vi "Map the Signals and Frames.vi"(8 "error in":errorcluster, 11 "References":T1) -> (0 "error out":errorcluster)   [LabVIEW 2025, in "CAN-LIN Raw Bus Capture UI.lvlib"]
uses:
  CAN-LIN Raw Bus Capture UI.lvlib
  <vilib>/xnet/xnet.llb/XNET Create Session (Conversion).vi
  <resource>/objmgr/xnet.rc
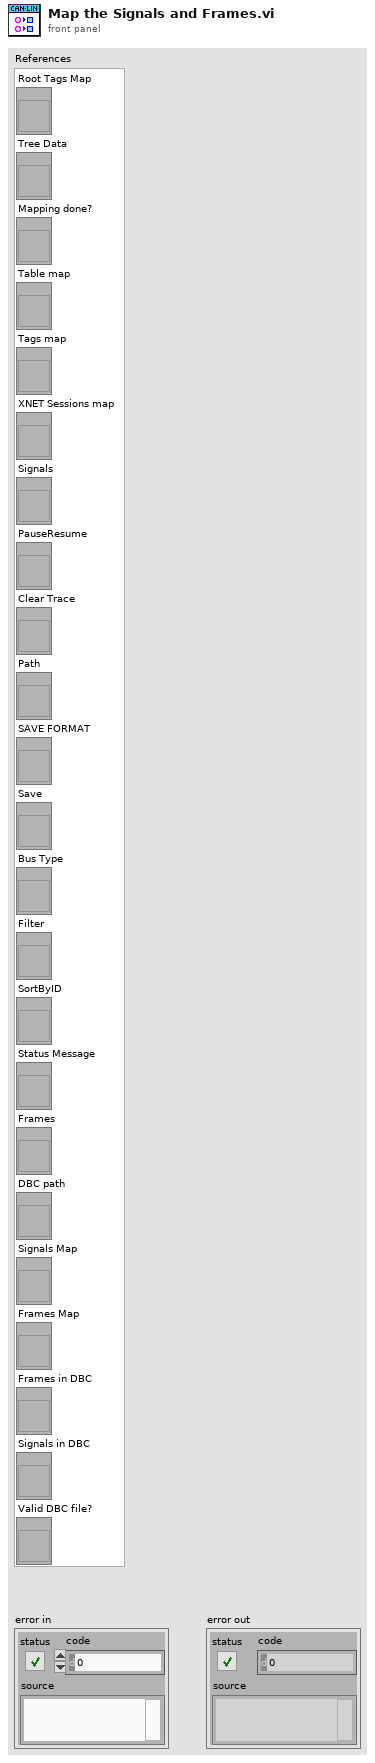
[diagram p1: front panel]
types:
  T1 = cluster{"Root Tags Map":refnum<vi>, "Tree Data":refnum<vi>, "Mapping done?":refnum<vi>, "Table map":refnum<vi>, "Tags map":refnum<vi>, "XNET Sessions map":refnum<vi>, "Signals":refnum<vi>, "PauseResume":refnum<vi>, "Clear Trace":refnum<vi>, "Path":refnum<vi>, "SAVE FORMAT":refnum<vi>, "Save":refnum<vi>, "Bus Type":refnum<vi>, "Filter":refnum<vi>, "SortByID":refnum<vi>, "Status Message":refnum<vi>, "Frames":refnum<vi>, "DBC path":refnum<vi>, "Signals Map":refnum<vi>, "Frames Map":refnum<vi>, "Frames in DBC":refnum<vi>, "Signals in DBC":refnum<vi>, "Valid DBC file?":refnum<vi>}
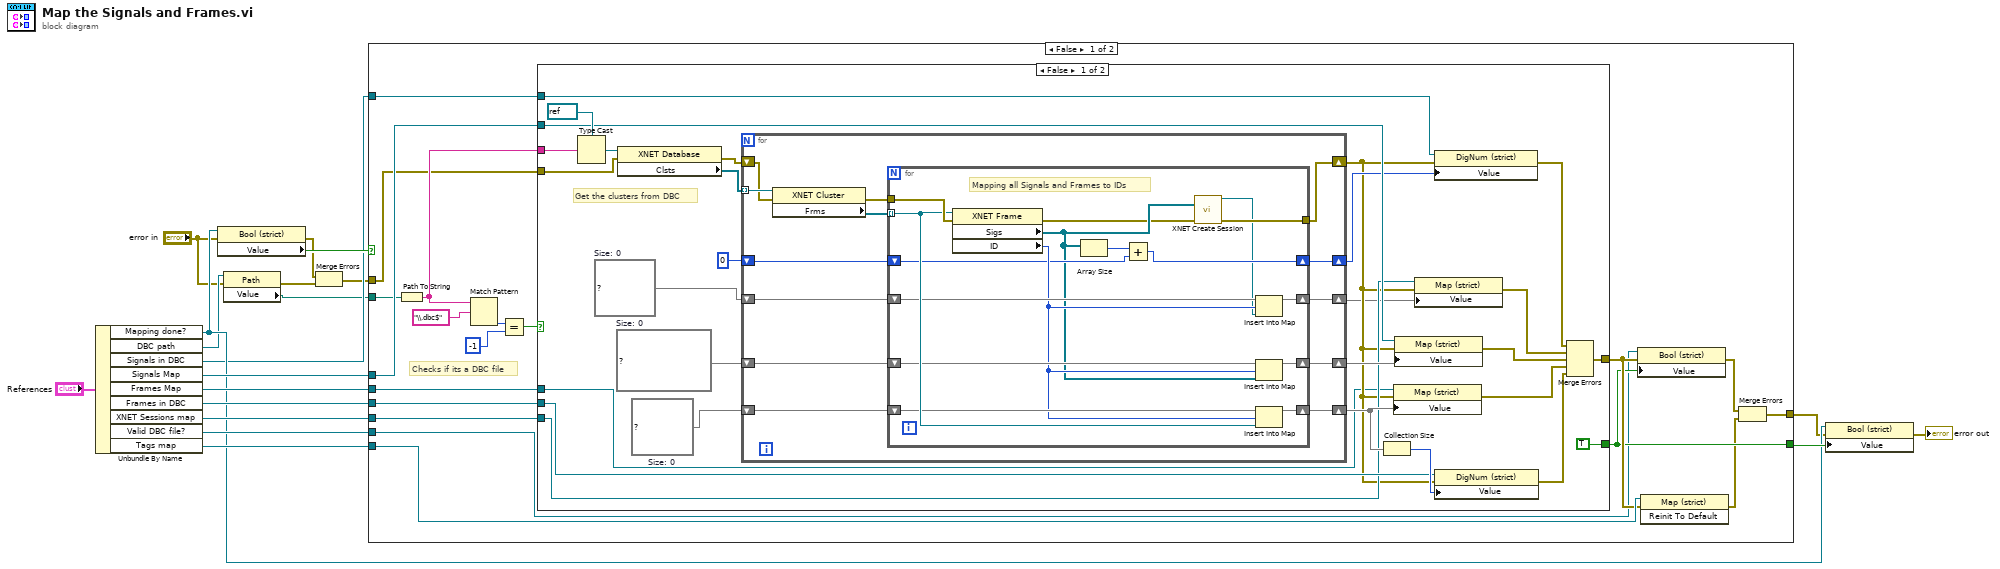
[diagram p0: block diagram]
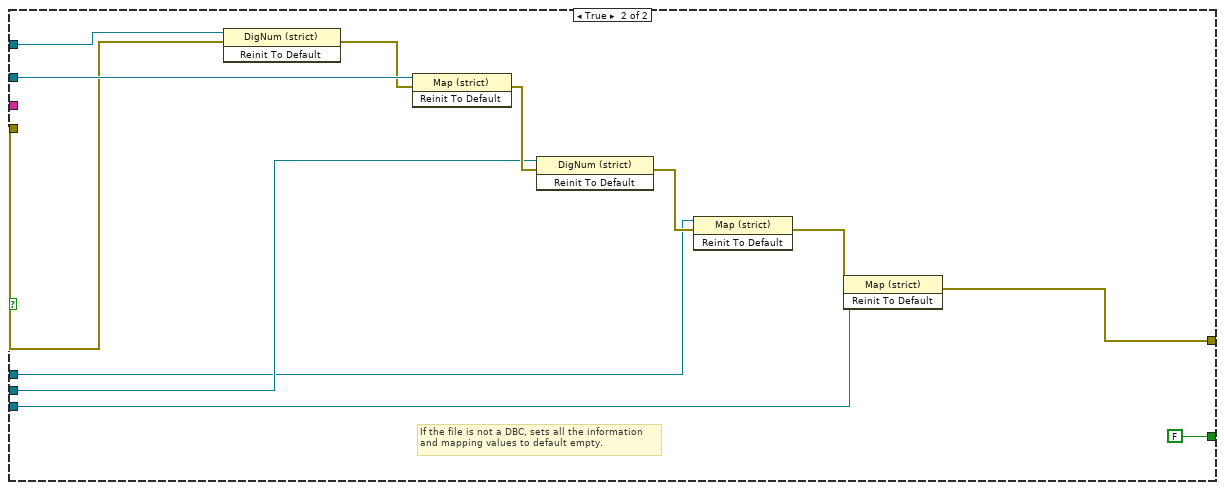
[diagram p2: hidden frame]
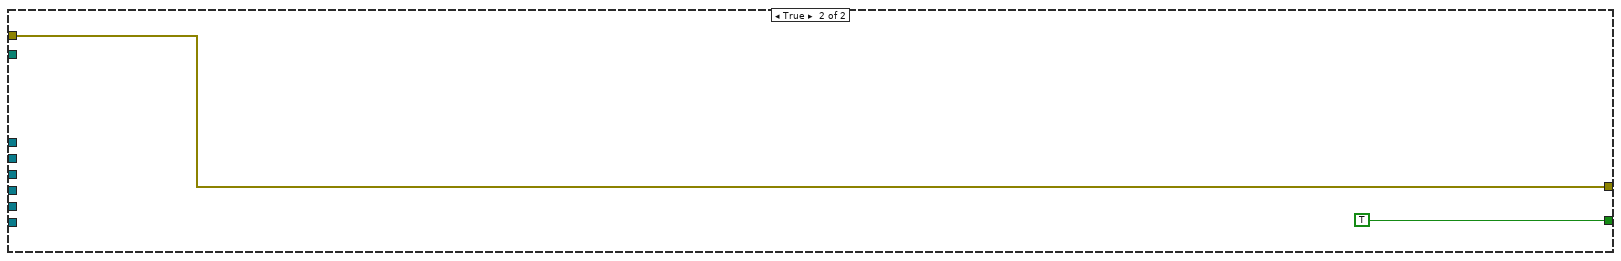
[diagram p3: hidden frame]
diagram:
  n1 = Unbundle By Name("References") -> ("Mapping done?"=w11:refnum<vi>, "DBC path"=w7:refnum<vi>, "Signals in DBC"=w8:refnum<vi>, "Signals Map"=w16:refnum<vi>, "Frames Map"=w19:refnum<vi>, "Frames in DBC"=w18:refnum<vi>, "XNET Sessions map"=w17:refnum<vi>, "Valid DBC file?"=w14:refnum<vi>, "Tags map"=w15:refnum<vi>)
  n2 = property class="Bool (strict)"(reference=w11, error in="error in") -> (error out=w3:errorcluster, "Value"=w13:bool)  [unwired: 1 out]
  n3 = property class="Path"(reference=w7, error in="error in") -> (error out=w5:errorcluster, "Value"=w2:path)  [unwired: 1 out]
  n4 = Merge Errors(w3, w5) -> (w4:errorcluster)
  n5 = case shown="False" w13 {
    tunnel: [w24 w108] -> w10
    tunnel: w4 -> [w20 w108]
    tunnel: [w27 TRUE ("Mapping done?")] -> w12
    tunnel: w19 -> [w37 _]
    tunnel: w16 -> [w38 _]
    tunnel: w18 -> [w31 _]
    tunnel: w8 -> [w30 _]
    tunnel: w17 -> [w23 _]
    tunnel: w14 -> [w22 _]
    tunnel: w15 -> [w29 _]
    tunnel: w2 -> [w21 _]
    frame False {
      # "Checks if its a DBC file"
      n6 = Path To String(path=w21) -> (string=w35:string)
      n7 = Match Pattern(string=w35, regular expression="\\.dbc$") -> (offset past match=w34:i32)  [unwired: 1 in, 3 out]
      n8 = Equal?(x=w34, y=-1) -> (x = y?=w32:bool)
      n9 = case shown="False" w32 {
        tunnel: w20 -> [w60 w100]
        tunnel: [TRUE ("Mapping done?") FALSE ("Mapping done?")] -> w27
        tunnel: w38 -> [w58 w102]
        tunnel: w37 -> [w39 w97]
        tunnel: [w55 w105] -> w28
        tunnel: w35 -> [w54 _]
        tunnel: w31 -> [w50 w98]
        tunnel: w30 -> [w46 w96]
        tunnel: w23 -> [w45 w106]
        frame False {
          w42 = map{u32, refnum<k21>} {}  # Size: 0
          w61 = map{u32, refnum<k21>} {}  # Size: 0
          w62 = map{u32, refnum<k21>[]} {}  # Size: 0
          # "Get the clusters from DBC"
          n10 = Type Cast(type=refnum<k21> refnum ("XNET Database"), x=w54) -> (*(type *) &x=w65:refnum<k21>)
          n11 = property class="XNET Database"(reference=w65, error in=w60) -> (error out=w66:errorcluster, "Clsts"=w64:refnum<k21>[])  [unwired: 1 out]
          n12 = for {
            tunnel: w64 -> [w79] mode=indexing
            shift-right: [w74] -> w52
            shift-left: w62 -> [w73]
            shift-right: [w72] -> w53
            shift-left: w61 -> [w71]
            shift-right: [w69] -> w47
            shift-left: 0 -> [w70]
            shift-right: [w75] -> w44
            shift-left: w66 -> [w77]
            shift-right: [w67] -> w40
            shift-left: w42 -> [w68]
            n13 = property class="XNET Cluster"(reference=w79, error in=w77) -> (error out=w76:errorcluster, "Frms"=w78:refnum<k21>[])  [unwired: 1 out]
            n14 = for {
              tunnel: w78 -> [w94] mode=indexing
              tunnel: w76 -> [w95]
              tunnel: [w81] -> w75
              shift-right: [w93] -> w74
              shift-left: w73 -> [w92]
              shift-right: [w91] -> w72
              shift-left: w71 -> [w90]
              shift-right: [w89] -> w69
              shift-left: w70 -> [w84]
              shift-right: [w87] -> w67
              shift-left: w68 -> [w88]
              # "Mapping all Signals and Frames to IDs"
              n15 = property class="XNET Frame"(reference=w94, error in=w95) -> (error out=w82:errorcluster, "Sigs"=w83:refnum<k21>[], "ID"=w86:u32)  [unwired: 1 out]
              n16 = Array Size(array=w83) -> (size(s)=w85:i32)
              n17 = Add(x=w85, y=w84) -> (x+y=w89:i32)
              n18 = call-poly <vilib>:"XNET Create Session.vi"("signal list"=w83, "error in (no error)"=w82) -> ("session out"=w80:refnum<k21>, "error out"=w81:errorcluster)  [unwired: 12 out]
              n19 = Insert Into Map(map in=w88, key=w86, value=w80) -> (map out=w87:map{u32, refnum<k21>})  [unwired: 2 out]
              n20 = Insert Into Map(map in=w92, key=w86, value=w83) -> (map out=w93:map{u32, refnum<k21>[]})  [unwired: 2 out]
              n21 = Insert Into Map(map in=w90, key=w86, value=w94) -> (map out=w91:map{u32, refnum<k21>})  [unwired: 2 out]
            }
          }
          n22 = Collection Size(1:w53) -> (0:w51:i32)
          n23 = property class="Map (strict)"(reference=w39, error in=w44, "Value"=w53) -> (error out=w56:errorcluster)  [unwired: 1 out]
          n24 = property class="Map (strict)"(reference=w58, error in=w44, "Value"=w52) -> (error out=w57:errorcluster)  [unwired: 1 out]
          n25 = property class="Map (strict)"(reference=w45, error in=w44, "Value"=w40) -> (error out=w43:errorcluster)  [unwired: 1 out]
          n26 = property class="DigNum (strict)"(reference=w46, error in=w44, "Value"=w47) -> (error out=w41:errorcluster)  [unwired: 1 out]
          n27 = property class="DigNum (strict)"(reference=w50, error in=w44, "Value"=w51) -> (error out=w49:errorcluster)  [unwired: 1 out]
          n28 = Merge Errors(w41, w43, w57, w56, w49) -> (w55:errorcluster)
        }
        frame True {
          # "If the file is not a DBC, sets all the information\nand mapping values to default empty."
          n29 = invoke class="DigNum (strict)" method="Reinit To Default"(reference=w96, error in=w100) -> (error out=w99:errorcluster)  [unwired: 1 in, 2 out]
          n30 = invoke class="Map (strict)" method="Reinit To Default"(reference=w102, error in=w99) -> (error out=w101:errorcluster)  [unwired: 1 in, 2 out]
          n31 = invoke class="DigNum (strict)" method="Reinit To Default"(reference=w98, error in=w101) -> (error out=w103:errorcluster)  [unwired: 1 in, 2 out]
          n32 = invoke class="Map (strict)" method="Reinit To Default"(reference=w97, error in=w103) -> (error out=w104:errorcluster)  [unwired: 1 in, 2 out]
          n33 = invoke class="Map (strict)" method="Reinit To Default"(reference=w106, error in=w104) -> (error out=w105:errorcluster)  [unwired: 1 in, 2 out]
        }
      }
      n34 = property class="Bool (strict)"(reference=w22, error in=w28, "Value"=w27) -> (error out=w25:errorcluster)  [unwired: 1 out]
      n35 = invoke class="Map (strict)" method="Reinit To Default"(reference=w29, error in=w28) -> (error out=w26:errorcluster)  [unwired: 1 in, 2 out]
      n36 = Merge Errors(w25, w26) -> (w24:errorcluster)
    }
    frame True {
    }
  }
  n37 = property class="Bool (strict)"(reference=w11, error in=w10, "Value"=w12) -> (error out=→"error out":errorcluster)  [unwired: 1 out]
